vi "20170509-lecture4-2 login.vi"() -> ()   [LabVIEW 2014]
panel:
  in  "stop":bool
  out "x .and. y?":bool
  in  "Passwords":string
  in  "Username":string
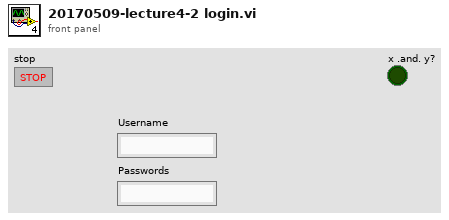
[diagram p1: front panel]
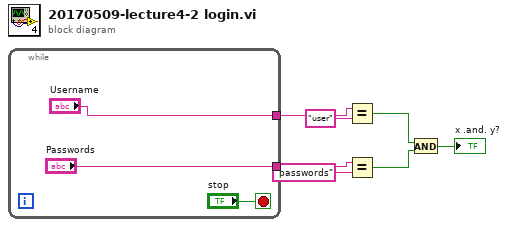
[diagram p0: block diagram]
diagram:
  n1 = while {
    tunnel: ["Passwords"] -> w5
    tunnel: ["Username"] -> w7
    stop <- "stop" stop-if-true
  }
  n2 = Equal?(x=w7, y="user") -> (x = y?=w3:bool)
  n3 = Equal?(x=w5, y="passwords") -> (x = y?=w2:bool)
  n4 = And(x=w3, y=w2) -> (x .and. y?=→"x .and. y?":bool)
